vi "clone.vi"(0 "reference":refnum<class "FinalStateNode.lvclass">, 5 "error in (no error)":errorcluster) -> (14 "reference out":refnum<class "FinalStateNode.lvclass">, 15 "clonedInterfaceNode":refnum<class "AbstractNode.lvclass">, 19 "error out":errorcluster)   [LabVIEW 2014, in "FinalStateNode.lvclass"]
doc: "public Object clone()"
uses:
  <resource>/Framework/Providers/Open_GDS/UML/FinalStateNode_class/FinalStateNode.lvclass
  <resource>/Framework/Providers/Open_GDS/UML/AbstractNode_class/AbstractNode.lvclass
  <resource>/Framework/Providers/Open_GDS/UML/MultiLineString_class/MultiLineString.lvclass
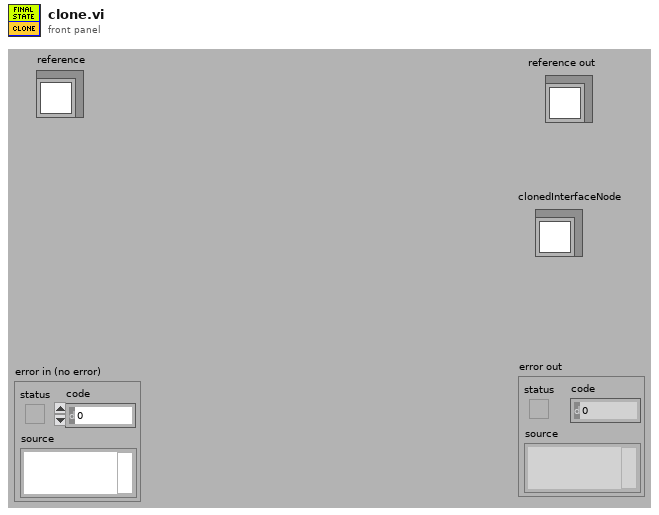
[diagram p1: front panel]
types:
  T1 = typedef "FinalStateNode.lvclass/ObjectAttributes.ctl" = cluster{"name":refnum<class "MultiLineString.lvclass">, "DEFAULT_WIDTH":i32, "DEFAULT_HEIGHT":i32}
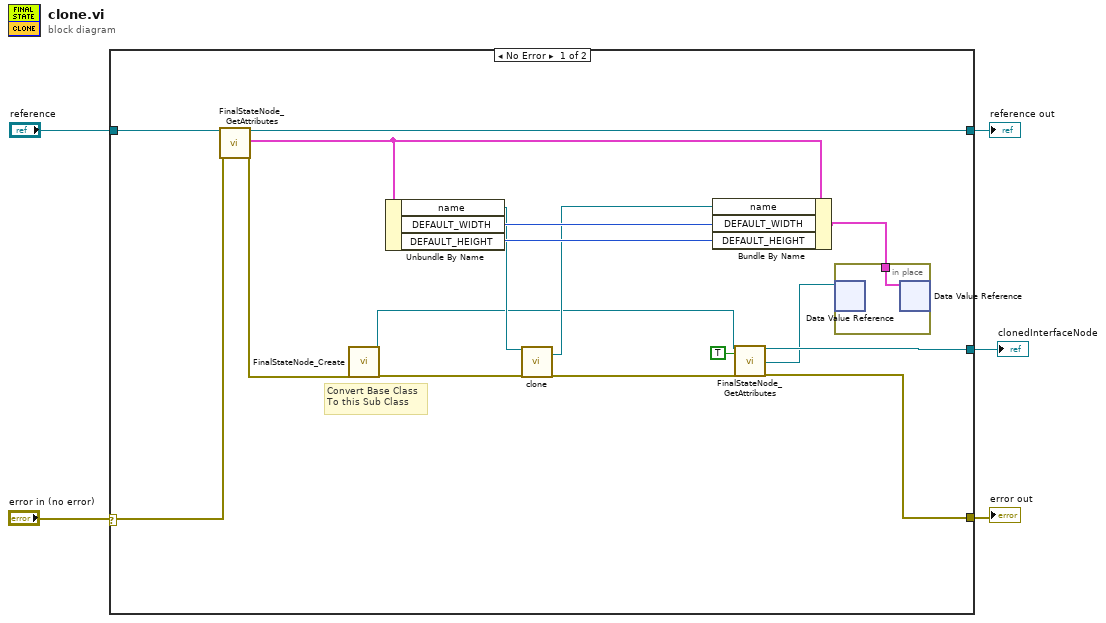
[diagram p0: block diagram]
diagram:
  n1 = case shown="No Error" "error in (no error)" {
    selector: "error in (no error)" -> [w21 w24]
    tunnel: "reference" -> [w22 w25]
    tunnel: [w8 w24] -> w4
    tunnel: [w13 w25] -> w3
    tunnel: [w9 _] -> w1
    frame No Error {
      # "Convert Base Class\nTo this Sub Class"
      n2 = call <resource>:"FinalStateNode_GetAttributes.vi"("reference in"=w22, "error in (no error)"=w21) -> ("reference out"=w13:refnum<class "FinalStateNode.lvclass">, "Data"=w10:T1, "error out"=w12:errorcluster)  [unwired: 1 in, 14 out]
      n3 = call <resource>:"FinalStateNode_Create.vi"("error in (no error)"=w12) -> ("reference out"=w14:refnum<class "FinalStateNode.lvclass">, "error out"=w18:errorcluster)  [unwired: 17 in]
      n4 = Unbundle By Name(w10) -> ("name"=w17:refnum<class "MultiLineString.lvclass">, "DEFAULT_WIDTH"=w20:i32, "DEFAULT_HEIGHT"=w19:i32)
      n5 = call-dynamic "clone.vi"("reference"=w17, "error in (no error)"=w18) -> ("clonedMultiLineString"=w16:refnum<class "MultiLineString.lvclass">, "error out"=w15:errorcluster)  [unwired: 15 in, 1 out]
      n6 = Bundle By Name(cluster=w10, "name"=w16, "DEFAULT_WIDTH"=w20, "DEFAULT_HEIGHT"=w19) -> (w6:T1)
      n7 = call <resource>:"FinalStateNode_GetAttributes.vi"("reference in"=w14, "OnlyGetDvrReference(False)"=TRUE, "error in (no error)"=w15) -> ("reference out"=w9:refnum<class "FinalStateNode.lvclass">, "DataRef"=w7:refnum<data-value>, "error out"=w8:errorcluster)  [unwired: 13 in, 1 out]
      n8 = in-place {
        in-place-border: w6 -> [w23]
        n9 = in-place-dvr #1(w7) -> ()  [unwired: 2 out]
        n10 = in-place-dvr #1(w23) -> ()  [unwired: 2 out]
      }
    }
    frame Error {
    }
  }
  "reference out" <- w3
  "error out" <- w4
  "clonedInterfaceNode" <- w1
